vi "Should Log Error.vi"(11 "error to report":errorcluster caption="报告的错误") -> (2 "Should Log Error?":bool caption="应记录错误？", 3 "dup error to report":errorcluster caption="报告的错误副本")   [LabVIEW 2013]
uses:
  Globals/Global - Configuration Options.vi
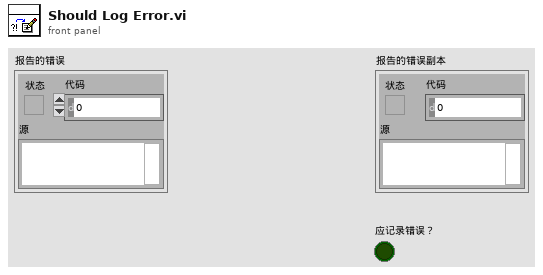
[diagram p1: front panel]
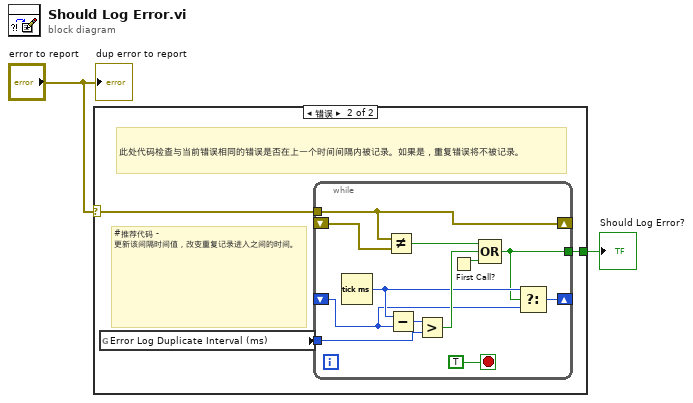
[diagram p0: block diagram]
diagram:
  n1 = case shown="错误" "error to report" {
    selector: "error to report" -> [_ w4]
    tunnel: [_ w5] -> w2
    frame No Error {
      # "不记录“无错误”"
    }
    frame Error {
      # "#推荐代码 - 更新该间隔时间值，改变重复记录进入之间的时间。"
      # "此处代码检查与当前错误相同的错误是否在上一个时间间隔内被记录。如果是，重复错误将不被记录。"
      n2 = global read "Global - Configuration Options.vi" "Error Log Duplicate Interval (ms)"() -> (w3:u32)
      n3 = while {
        tunnel: w4 -> [w16]
        shift-right: [w16] -> _
        shift-left: _ -> [w17]
        shift-right: [w7] -> _
        shift-left: _ -> [w8]
        tunnel: w3 -> [w14]
        tunnel: [w6] -> w5
        stop <- TRUE stop-if-true
        n4 = Tick Count (ms)() -> (millisecond timer value=w9:u32)
        n5 = Not Equal?(x=w16, y=w17) -> (x != y?=w12:bool)
        n6 = Subtract(x=w9, y=w8) -> (x-y=w15:u32)
        n7 = Greater?(x=w15, y=w14) -> (0:w11:bool)
        n8 = First Call?() -> (First Call?: T/F=w10:bool)
        n9 = Compound Arithmetic op=OR(w12, w11, w10) -> (w6:bool)
        n10 = Select(t=w9, s=w6, f=w8) -> (s? t:f=w7:u32)
      }
    }
  }
  "Should Log Error?" <- w2
  "dup error to report" <- "error to report"
